vi "Load Step Config Class.vi"(8 "error in (no error)":errorcluster, 11 "Step Folder Path":path) -> (0 "error out":errorcluster, 3 "Step Config out":refnum<class "Step Config.lvclass">)   [LabVIEW 2015, in "Configuration Tool.lvlib"]
uses:
  Configuration Tool.lvlib
  Prototype/classes/Step/Config/Step Config.lvclass
  <vilib>/Utility/error.llb/Error Cluster From Error Code.vi
  <vilib>/ErrorRing/Error Ring.xnode
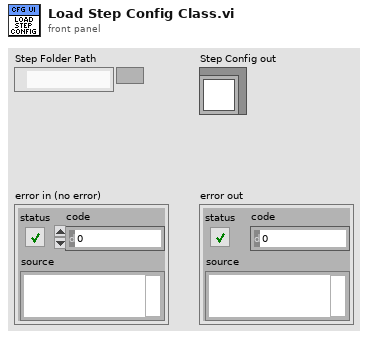
[diagram p1: front panel]
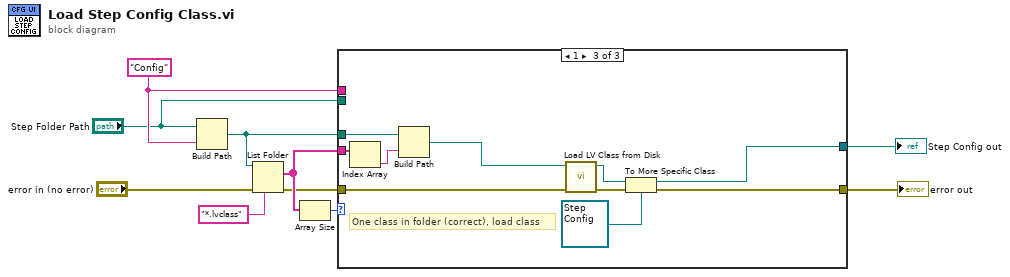
[diagram p0: block diagram]
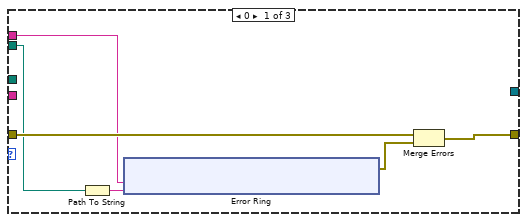
[diagram p2: hidden frame]
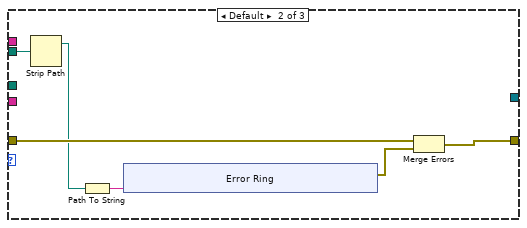
[diagram p3: hidden frame]
diagram:
  w10 = "Config" ("name or relative path")
  n1 = Build Path(base path="Step Folder Path", name or relative path=w10) -> (appended path=w4:path)
  n2 = List Folder(path=w4, pattern="*.lvclass", error in="error in (no error)") -> (filenames=w6:string[], error out=w2:errorcluster)  [unwired: 1 in, 2 out]
  n3 = Array Size(array=w6) -> (size(s)=w7:i32)
  n4 = case shown="1" w7 {
    tunnel: w2 -> [w16 w30 w44]
    tunnel: w4 -> [_ _ w43]
    tunnel: w6 -> [_ _ w42]
    tunnel: [w15 w29 w41] -> w5
    tunnel: "Step Folder Path" -> [w14 w28 _]
    tunnel: [_ _ w40] -> w9
    tunnel: w10 -> [w11 _ _]
    frame 0 {
      n5 = Path To String(path=w14) -> (string=w12:string)
      n6 = xnode "Error Ring"("parameter 0"=w11, "parameter 1"=w12) -> ("error out"=w13:errorcluster)
      n7 = Merge Errors(w16, w13) -> (w15:errorcluster)
    }
    frame Default {
      n8 = Strip Path(path=w28) -> (stripped path=w27:path)  [unwired: 1 out]
      n9 = Path To String(path=w27) -> (string=w26:string)
      n10 = xnode "Error Ring"("parameter 0"=w26) -> ("error out"=w25:errorcluster)
      n11 = Merge Errors(w30, w25) -> (w29:errorcluster)
    }
    frame 1 {
      # "One class in folder (correct), load class"
      n12 = Index Array(array=w42) -> (element=w39:string)  [unwired: 1 in]
      n13 = Build Path(base path=w43, name or relative path=w39) -> (appended path=w38:path)
      n14 = call "Load LV Class from Disk.vi"("error in"=w44, "Class Path"=w38) -> ("error out"=w45:errorcluster, "Object Out"=w47:refnum<class>)  [unwired: 8 in]
      n15 = To More Specific Class(target class=refnum<class "Step Config.lvclass"> refnum ("Step Config.lvclass"), reference=w47, error in=w45) -> (specific class reference=w40:refnum<class "Step Config.lvclass">, error out=w41:errorcluster)
    }
  }
  "Step Config out" <- w9
  "error out" <- w5
